vi "WinCI Get Command Options.vi"(7 "advanced options in":variant, 8 "error in (no error)":errorcluster, 10 "interface command":T1 items=["GET", "CHECKOUT", "CHECKIN", "UNCHECKOUT", "ADD", "REMOVE", "DIFF", "HISTORY", "RENAME", "PROPERTIES", "OPTIONS"], 11 "source control reference in":T2) -> (0 "error out":errorcluster, 1 "dialog box cancelled?":bool, 2 "status message":string, 3 "source control reference out":T2, 5 "advanced options out":variant)   [LabVIEW 2017, in "NI_SCC_WinCI.lvlib"]
uses:
  <vilib>/SourceControl/Providers/WinCI/NI_SCC_WinCI.lvlib
  <vilib>/SourceControl/sccapi/SCCAPI Refnum.ctl
  <vilib>/SourceControl/Providers/WinCI/WinCI Interface Command.ctl
  <vilib>/SourceControl/support/SCCSup Message Strings GLBL.vi
  <vilib>/SourceControl/sccapi/NI_SCC.lvlib
panel:
  out "result":i32
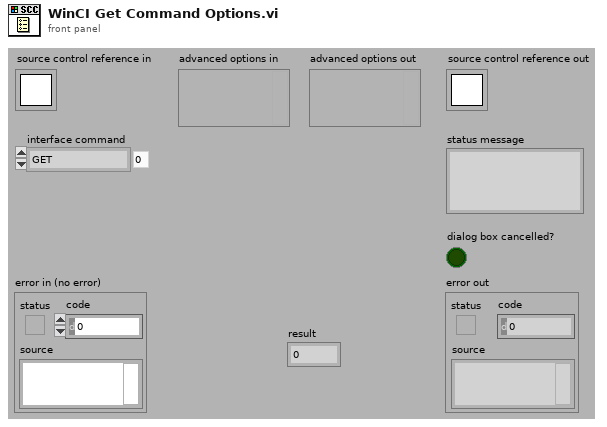
[diagram p1: front panel]
types:
  T1 = typedef "NI_SCC_WinCI.lvlib/WinCI Interface Command.ctl" = i32
  T2 = typedef "NI_SCC.lvlib/SCCAPI Refnum.ctl" = refnum<k1>
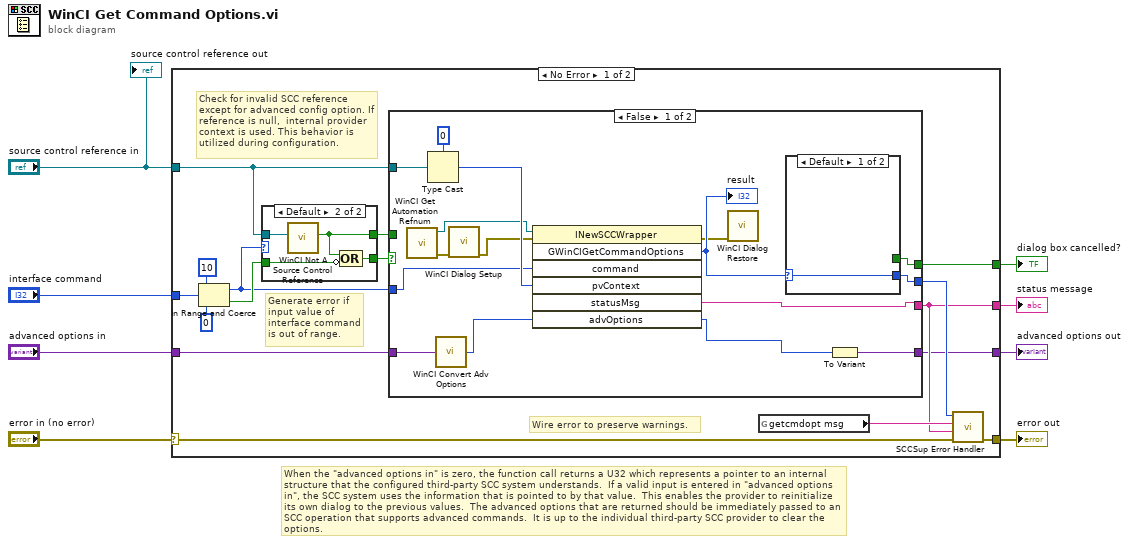
[diagram p0: block diagram]
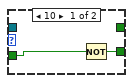
[diagram p2: hidden frame]
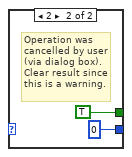
[diagram p3: hidden frame]
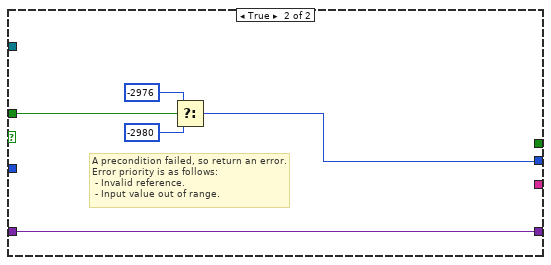
[diagram p4: hidden frame]
diagram:
  # "When the \"advanced options in\" is zero, the function call returns a U32 which represents a pointer to an internal structure that the configured third-party SCC system understands.  If a valid input is entered in \"advanced options in\", the SCC system uses the information that is pointed to by that value.  This enables the provider to reinitialize its own dialog to the previous values.  The advanced options that are returned should be immediately passed to an SCC operation that supports advanced commands.  It is up to the individual third-party SCC provider to clear the options."
  n1 = case shown="No Error" "error in (no error)" {
    selector: "error in (no error)" -> [w16 w56]
    tunnel: [w24 w56] -> w7
    tunnel: "source control reference in" -> [w17 _]
    tunnel: [w21 _] -> w5
    tunnel: "interface command" -> [w18 _]
    tunnel: [w15 _] -> w3
    tunnel: "advanced options in" -> [w11 w55]
    tunnel: [w10 w55] -> w1
    frame No Error {
      # "Check for invalid SCC reference except for advanced config option. If reference is null,  internal provider context is used. This behavior is utilized during configuration."
      # "Generate error if input value of interface command  is out of range."
      # "Wire error to preserve warnings."
      n2 = In Range and Coerce(upper limit=10, x=w18, lower limit=0) -> (coerced(x)=w9:T1, In Range?=w12:bool)
      n3 = case shown="Default" w9 {
        tunnel: w17 -> [_ w28]
        tunnel: [w25 w30] -> w14
        tunnel: [_ w27] -> w13
        tunnel: w12 -> [w26 w29]
        frame 10 {
          n4 = Not(x=w26) -> (.not. x?=w25:bool)
        }
        frame Default {
          n5 = call <vilib>:"WinCI Not A Source Control Reference.vi"("source control reference in"=w28) -> ("not a source control reference?"=w27:bool)  [unwired: 1 in, 9 out]
          n6 = Compound Arithmetic op=OR(w27, invert w29) -> (w30:bool)
        }
      }
      n7 = case shown="False" w14 {
        tunnel: w17 -> [w46 _]
        tunnel: w9 -> [w36 _]
        tunnel: [w44 w51] -> w23
        tunnel: [w38 _] -> w21
        tunnel: [w43 _] -> w15
        tunnel: w13 -> [_ w54]
        tunnel: w11 -> [w41 w50]
        tunnel: [w42 w50] -> w10
        frame False {
          n8 = call <vilib>:"WinCI Get Automation Refnum.vi"() -> ("error out"=w33:errorcluster, "automation refnum"=w35:refnum<k7>)  [unwired: 10 out]
          n9 = Type Cast(type=u32 0, x=w46) -> (*(type *) &x=w37:u32)
          n10 = call <vilib>:"WinCI Convert Adv Options.vi"("advanced options"=w41) -> ("command options"=w40:u32)  [unwired: 4 out]
          n11 = call <vilib>:"WinCI Dialog Setup.vi"("error in"=w33) -> ("error out"=w32:errorcluster)  [unwired: 10 out]
          n12 = invoke class="INewSCCWrapper" method="GWinCIGetCommandOptions"(reference=w35, error in=w32, "command"=w36, "pvContext"=w37, "advOptions"=w40) -> (error out=w31:errorcluster, "GWinCIGetCommandOptions"=w34:i32, "statusMsg"=w38:string, "advOptions"=w39:u32)  [unwired: 2 in, 3 out]
          "result" <- w34
          n13 = call <vilib>:"WinCI Dialog Restore.vi"("error in"=w31) -> ()  [unwired: 11 out]
          n14 = case shown="Default" w34 {
            selector: w34 -> [w47 _]
            tunnel: [w47 0 ("result")] -> w44
            tunnel: [_ TRUE] -> w43
            frame Default {
            }
            frame 2 {
              # "Operation was cancelled by user (via dialog box).  Clear result since this is a warning."
            }
          }
          n15 = To Variant(anything=w39) -> (Variant=w42:variant)
        }
        frame True {
          # "A precondition failed, so return an error. \nError priority is as follows:\n - Invalid reference.  \n - Input value out of range."
          n16 = Select(t=-2976 ("result"), s=w54, f=-2980) -> (s? t:f=w51:i32)
        }
      }
      n17 = global read "SCCSup Message Strings GLBL.vi" "getcmdopt msg"() -> (w22:string)
      n18 = call <vilib>:"SCCSup Error Handler.vi"("error in (no error)"=w16, "additional message"=w21, "operation message"=w22, "scc error code"=w23) -> ("error out"=w24:errorcluster)  [unwired: 7 out]
    }
    frame Error {
    }
  }
  "error out" <- w7
  "status message" <- w5
  "dialog box cancelled?" <- w3
  "advanced options out" <- w1
  "source control reference out" <- "source control reference in"
